vi "rm.server.get reserver.vi"(8 "error in (no error)":errorcluster, 10 "Name in Bitfile":string, 11 "Item Ref in":T1 format="%.0x") -> (0 "error out":errorcluster, 1 "found?":bool, 2 "Reserver Node Ref":T1=18446744073709551615 format="%.0x", 3 "Item Ref out":T1 format="%.0x")   [LabVIEW 2016, in "RM.Server.lvlib"]
uses:
  RM.Server.lvlib
  <vilib>/NI Veristand/Custom Device API/Custom Device Item Ref.ctl
  <vilib>/NI Veristand/Custom Device API/Get Item Property (Dependent Node Pointer).vi
  <vilib>/NI VeriStand/Custom Device API/Custom Device API.lvlib
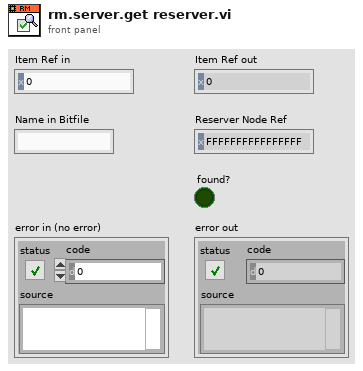
[diagram p1: front panel]
types:
  T1 = typedef "Custom Device API.lvlib/Custom Device Item Ref.ctl" = u64
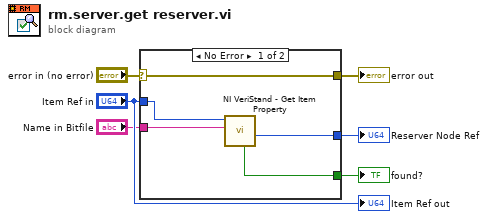
[diagram p0: block diagram]
diagram:
  n1 = case shown="No Error" "error in (no error)" {
    selector: "error in (no error)" -> [w11 w12]
    tunnel: [w11 w12] -> w5
    tunnel: "Item Ref in" -> [w10 _]
    tunnel: "Name in Bitfile" -> [w9 _]
    tunnel: [w8 _] -> w2
    tunnel: [w7 _] -> w1
    frame No Error {
      n2 = call-poly <vilib>:"NI VeriStand - Get Item Property.vi"("Property Name"=w9, "Item Ref in"=w10) -> ("Dependent Node Ref"=w7:T1, "Found"=w8:bool)  [unwired: 6 in, 2 out]
    }
    frame Error {
    }
  }
  "error out" <- w5
  "found?" <- w2
  "Reserver Node Ref" <- w1
  "Item Ref out" <- "Item Ref in"
